vi "Read AI DAQ_MCC_HiSpd.vi"(8 "error in (no error)":errorcluster, 10 "MeasSettings":T1={"Data Rate 9775"=3.0, "Data Rate 9215"=1200000.0, "Samples RMS 9215"=480000, "Samples RMS 9775"=3}, 11 "BoardNum":u32) -> (0 "error out":errorcluster, 2 "Start time":timestamp, 3 "AI Data[]":dbl[](array[numeric]))   [LabVIEW 2019, in "DAQ_Engine.lvclass"]
doc: "Developed by Kevin Thompson\nkevin@thompsonengineering.net\n\nCopyright 2020\nThompson Engineering, LLC"
uses:
  DAQ_Engine.lvclass
  support/DAQ Lib/ToEng(array).vi
  Common/DataTypes/Measurement Config--cluster.ctl
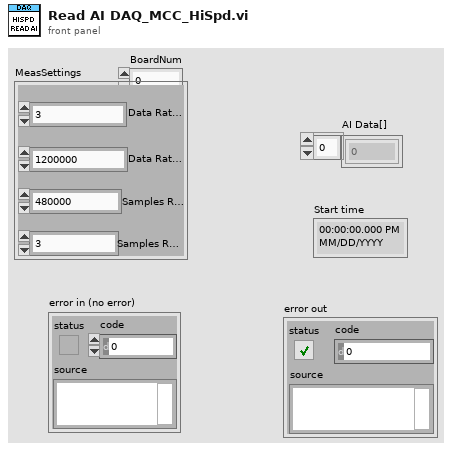
[diagram p1: front panel]
types:
  T1 = typedef "Measurement Config--cluster.ctl" = cluster{"Data Rate 9775":dbl, "Data Rate 9215":dbl, "Samples RMS 9215":u32, "Samples RMS 9775":u32}
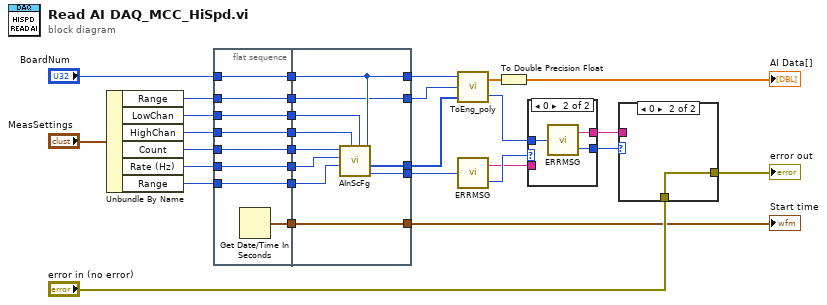
[diagram p0: block diagram]
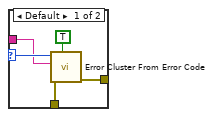
[diagram p3: hidden frame]
diagram:
  n1 = Unbundle By Name("MeasSettings") -> ("Range"=w25:i32, "LowChan"=w26:i32, "HighChan"=w30:i32, "Count"=w27:i32, "Rate (Hz)"=w28:i32, "Range"=w29:i32)
  n2 = flat-sequence {
    tunnel: w30 -> [w38]
    tunnel: [w38] -> w22
    tunnel: [w37] -> w21
    tunnel: w29 -> [w36]
    tunnel: [w36] -> w20
    tunnel: w28 -> [w35]
    tunnel: [w35] -> w19
    tunnel: w27 -> [w34]
    tunnel: [w34] -> w18
    tunnel: w26 -> [w33]
    tunnel: [w33] -> w17
    tunnel: [w32] -> w16
    tunnel: "BoardNum" -> [w32]
    tunnel: [w31] -> w15
    tunnel: w25 -> [w31]
    tunnel: [w48] -> w14
    tunnel: [w46] -> w13
    tunnel: w22 -> [w47]
    tunnel: [w45] -> w1
    tunnel: w21 -> [w45]
    tunnel: w20 -> [w44]
    tunnel: w19 -> [w43]
    tunnel: w18 -> [w42]
    tunnel: w17 -> [w41]
    tunnel: w16 -> [w40]
    tunnel: [w40] -> w12
    tunnel: [w39] -> w11
    tunnel: w15 -> [w39]
    frame #0 {
      n3 = Get Date/Time In Seconds() -> (seconds since 1Jan1904=w37:timestamp)
    }
    frame #1 {
      n4 = call "AInScFg.VI"("BoardNum"=w40, "LowChan"=w41, "HighChan"=w47, "Range"=w44, "Rate"=w43, "Count"=w42) -> ("ErrCode"=w48:i32, "ADData"=w46:u16[])  [unwired: 2 in, 1 out]
    }
  }
  n5 = call-poly "ToEng_poly.VI"("AD Data"=w13, "Range"=w11, "BoardNum"=w12) -> ("ErrCode"=w7:i32, "Eng Units"=w10:sgl[])
  n6 = call "ERRMSG.VI"("ErrCode"=w14) -> ("ErrMsg"=w8:string, "ErrCode (Out)"=w9:i32)
  n7 = To Double Precision Float(number=w10) -> (double precision float=→"AI Data[]":dbl[])
  n8 = case shown="0" w9 {
    selector: w9 -> [w50 _]
    tunnel: w7 -> [_ w53]
    tunnel: [w50 w52] -> w24
    tunnel: w8 -> [w49 _]
    tunnel: [w49 w51] -> w23
    frame Default {
    }
    frame 0 {
      n9 = call "ERRMSG.VI"("ErrCode"=w53) -> ("ErrMsg"=w51:string, "ErrCode (Out)"=w52:i32)
    }
  }
  n10 = case shown="0" w24 {
    selector: w24 -> [w57 _]
    tunnel: [w58 w59] -> w4
    tunnel: w23 -> [w56 _]
    tunnel: "error in (no error)" -> [w55 w59]
    frame Default {
      n11 = call <vilib>:"Error Cluster From Error Code.vi"("show call chain? (False)"=TRUE, "error in (no error)"=w55, "error message (\"\")"=w56, "error code (0)"=w57) -> ("error out"=w58:errorcluster)  [unwired: 5 in]
    }
    frame 0 {
    }
  }
  "error out" <- w4
  "Start time" <- w1
